vi "Prepare Results.vi"(8 "error in (no error)":errorcluster, 9 "Execution Time":dbl, 11 "LUnit Test Case In":refnum<class "LUnit Test Case.lvclass">) -> (0 "error out":errorcluster, 2 "Results":T1[](array[typedef]), 3 "LUnit Test Case Out":refnum<class "LUnit Test Case.lvclass">)   [LabVIEW 2020, in "LUnit Test Case.lvclass"]
uses:
  LUnit Test Case.lvclass
  Core/Result/Result.ctl
  Core/Result/Status.ctl
  Core/Result/Type.ctl
  LUnit Test Case.lvclass/LUnit Test Case.ctl
  Core/Result/Result.lvlib
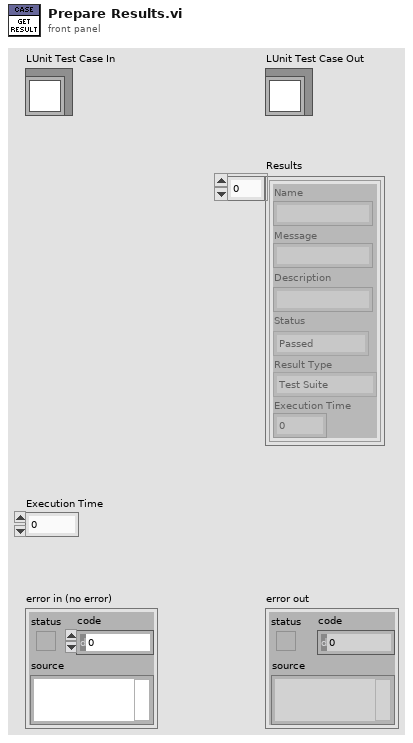
[diagram p1: front panel]
types:
  T1 = typedef "Result.lvlib/Result.ctl" = cluster{"Name":string, "Message":string, "Description":string, "Status":T2, "Result Type":T3, "Execution Time":dbl}
  T2 = typedef "Result.lvlib/Status.ctl" = enum16{"", "Passed", "Failed", "Error", "Skipped", "Setup Error", "Broken", "Teardown Error"}
  T3 = typedef "Result.lvlib/Type.ctl" = enum16{"Test Case", "Test Suite", "Test Run", "Pass", "Fail", "Skip", "Pass if", "Fail if", "Pass if Error", "Fail if Error", "Pass if Equal", "Fail if Equal"}
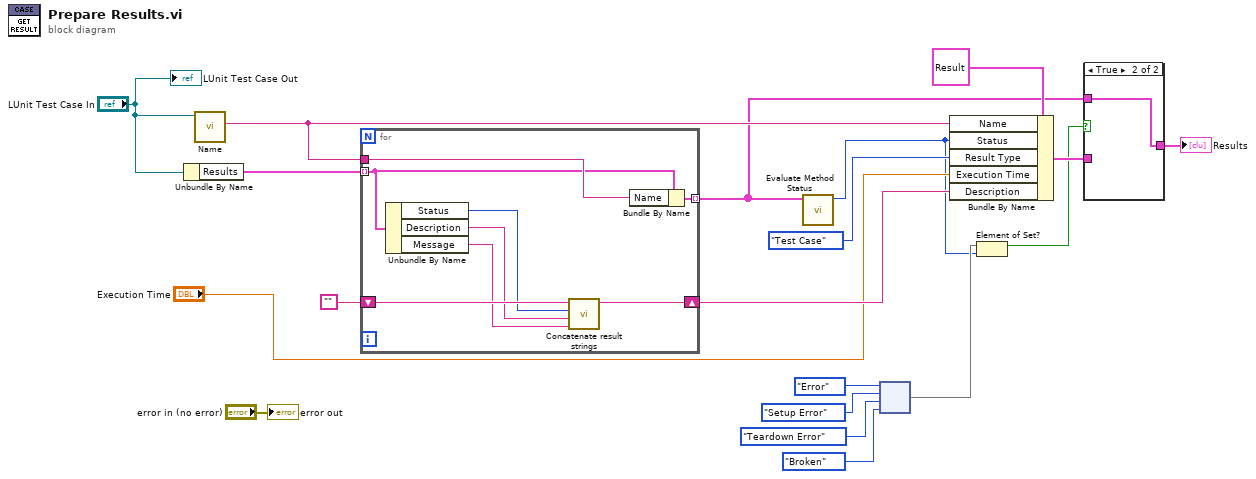
[diagram p0: block diagram]
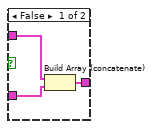
[diagram p2: hidden frame]
diagram:
  n1 = Unbundle By Name("LUnit Test Case In") -> ("Results"=w18:T1[])
  n2 = call-dynamic "Name.vi"("LUnit Test Case in"="LUnit Test Case In") -> ("Name"=w16:string)  [unwired: 8 in, 2 out]
  n3 = for {
    tunnel: w18 -> [w24] mode=indexing
    tunnel: w16 -> [w27]
    tunnel: [w26] -> w14 mode=indexing
    shift-right: [w20] -> w9
    shift-left: "" ("Input String") -> [w25]
    n4 = Unbundle By Name(w24) -> ("Status"=w23:T2, "Description"=w22:string, "Message"=w21:string)
    n5 = call "Concatenate result strings.vi"("Message"=w21, "Description"=w22, "Status"=w23, "Input String"=w25) -> ("Output String"=w20:string)  [unwired: 7 in]
    n6 = Bundle By Name(cluster=w24, "Name"=w27) -> (w26:T1)
  }
  n7 = call "Evaluate Method Status.vi"("Results"=w14) -> ("Status"=w2:T2)  [unwired: 10 in]
  n8 = node(Status."Error" ("Status"), Status."Setup Error" ("Status"), Status."Teardown Error" ("Status"), Status."Broken" ("Status")) -> (w3:set{T2})
  n9 = Bundle By Name(cluster=T1 {"Name"="", "Message"="", "Description"="", "Status"=enum."Passed", "Result Type"=enum."Test Case", "Execution Time"=0.0} ("Results"), "Name"=w16, "Status"=w2, "Result Type"=Type."Test Case", "Execution Time"="Execution Time", "Description"=w9) -> (w12:T1)
  n10 = Element of Set?(10:w2, 11:w3) -> (3:w1:bool)
  n11 = case shown="True" w1 {
    tunnel: w14 -> [w30 w31]
    tunnel: [w29 w31] -> w13
    tunnel: w12 -> [w28 _]
    frame False {
      n12 = Build Array (concatenate)(w30, w28) -> (w29:T1[])
    }
    frame True {
    }
  }
  "Results" <- w13
  "error out" <- "error in (no error)"
  "LUnit Test Case Out" <- "LUnit Test Case In"
